vi "Read Filament Heater ADC.vi"() -> (0 "Heater 4":dbl caption="Heater 1", 1 "Heater 3":dbl caption="Heater 1", 2 "Heater 2":dbl caption="Heater 1", 3 "Heater 1":dbl)   [LabVIEW 2018]
uses:
  Type/_RT Command.ctl
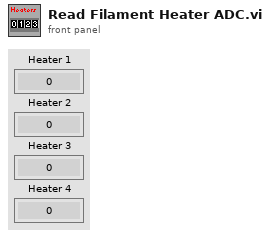
[diagram p1: front panel]
types:
  T1 = typedef "_RT Command.ctl" = enum16{"xml Start Run", "xml Start Actual Run", "xml Stop Run", "xml Runtime Update", "xml Get Status", "xml Get Table", "xml Set Table", "xml Get Configuration", "xml System Status", "xml Set LC Input Logic", "xml Get Data", "xml Get Info", "Start", "StartActualRun", "Stop", "Runtime Update", "Get Data", "Get Info", "Get Status", "Get Param", "Get Config", "Get Table", "Read ADC", "Set Oscillator", "Update Config", "Update Table", "Set All Pol", "Set Pol and DC", "Set Max Mass", "Toggle RP", "Toggle EL", "Set PIC", "Initialize Turbo", "Send Turbo Comm", "Close Turbo", "P1", "P2", "P3", "Send Serial", "Set LC Out", "Get LC In", "Read VAC", "Test Table", "Toggle Power", "Get Startup", "Set Startup", "Get ADC Table", "Set ADC Table", "Get Brief Status", "Get Detail Status", "Auxiliary Update", "Set CC Logics", "Set CC Input Logics", "Ignore Error", "invalid"}
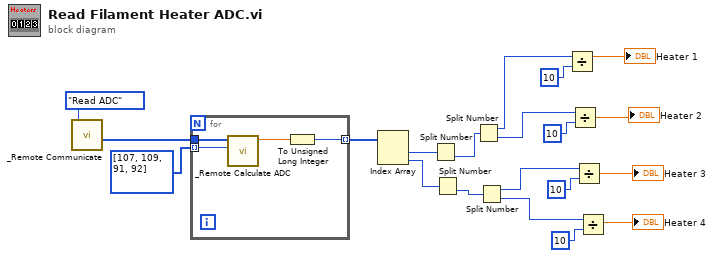
[diagram p0: block diagram]
diagram:
  n1 = call "_Remote Communicate.vi"("Command"=_RT_Command."Read ADC") -> ("Data Array"=w19:i32[])  [unwired: 5 in, 3 out]
  n2 = for {
    tunnel: w19 -> [w24]
    tunnel: u8[] [107, 109, 91, 92] ("ADC Channel (64)") -> [w23] mode=indexing
    tunnel: [w21] -> w17 mode=indexing
    n3 = call "_Remote Calculate ADC.vi"("ADC Channel (64)"=w23, "ADC Values"=w24) -> ("Raw Reading"=w22:dbl)  [unwired: 3 in, 2 out]
    n4 = To Unsigned Long Integer(number=w22) -> (unsigned 32bit integer=w21:u32)
  }
  n5 = Index Array(array=w17) -> (element #1=w16:u32, element #2=w15:u32)  [unwired: 2 in]
  n6 = Split Number(x=w16) -> (lo(x)=w14:u16)  [unwired: 1 out]
  n7 = Split Number(x=w15) -> (lo(x)=w13:u16)  [unwired: 1 out]
  n8 = Split Number(x=w14) -> (hi(x)=w12:u8, lo(x)=w6:u8)
  n9 = Split Number(x=w13) -> (hi(x)=w5:u8, lo(x)=w4:u8)
  n10 = Divide(x=w12, y=u8 10) -> (x/y=→"Heater 1":dbl)
  n11 = Divide(x=w6, y=u8 10) -> (x/y=→"Heater 2":dbl)
  n12 = Divide(x=w5, y=u8 10) -> (x/y=→"Heater 3":dbl)
  n13 = Divide(x=w4, y=u8 10) -> (x/y=→"Heater 4":dbl)
